vi "PrimeMode API.vi"(8 "error in (no error)":errorcluster, 10 "Pre Purge API Data":T1={"Interval (s)"=0.1, "PurgeDuration (s)"=0.1, "Repeats"=0, "PrimingMode"=enum."Pre-Purge", "Head"=enum."1"}, 11 "TopLevel in":refnum<class "TopLevel.lvclass">) -> (0 "error out":errorcluster, 3 "TopLevel out":refnum<class "TopLevel.lvclass">)   [LabVIEW 2022 SP3, in "TopLevel.lvclass"]
uses:
  TopLevel.lvclass
  Typedefs/PrimingMode APIData.ctl
  Typedefs/PurgeMode--Enum.ctl
  Typedefs/PrinterHeads--Enum.ctl
  Typedefs/API Command Cluster.ctl
  Typedefs/API Command Enum.ctl
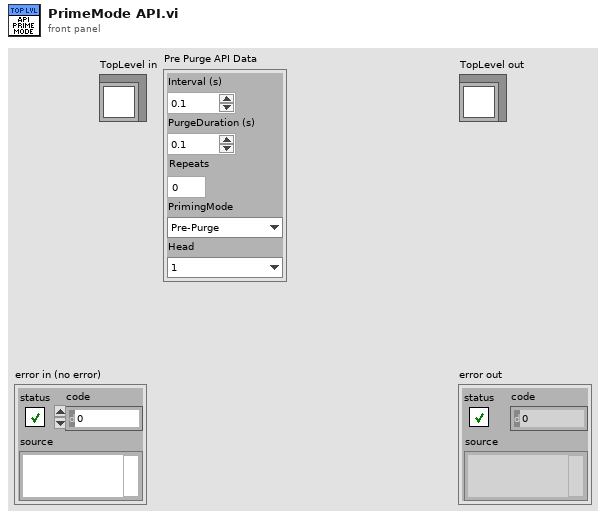
[diagram p1: front panel]
types:
  T1 = typedef "TopLevel.lvclass/PrimingMode APIData.ctl" = cluster{"Interval (s)":dbl, "PurgeDuration (s)":dbl, "Repeats":u8, "PrimingMode":T2, "Head":T3}
  T2 = typedef "PurgeMode--Enum.ctl" = enum16{"Pre-Purge", "Purge", "Spit", "Prime"}
  T3 = typedef "PrinterHeads--Enum.ctl" = enum16{"1", "2", "3", "4", "5", "6", "-1"}
  T4 = typedef "TopLevel.lvclass/API Command Enum.ctl" = enum16{"Execute Printer Commands", "Pre Purge", "Enable Ink Ch-1", "Enable Ink Ch-2", "Enable Ink Ch-3", "Enable Ink Ch-4", "Enable Ink Ch-5", "Enable Ink Ch-6", "Disable Ink Ch-1", "Disable Ink Ch-2", "Disable Ink Ch-3", "Disable Ink Ch-4", "Disable Ink Ch-5", "Disable Ink Ch-6", "ExecuteIdlePrintCycle", "StopIdlePrintCycle", "Abort", "LoadDLP2GUIConfig", "SaveDLP2GUIConfig", "PrimingMode", "SetHeadTemperature", "EnableHead", "EnableHeadHeat", "SetSystemMode", "HeadPrint"}
  T5 = typedef "TopLevel.lvclass/API Command Cluster.ctl" = cluster{"Command":T4, "Arguments":string, "Data":variant}
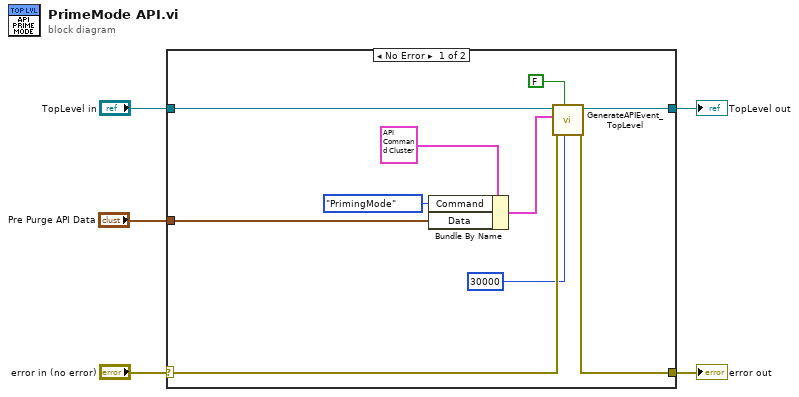
[diagram p0: block diagram]
diagram:
  n1 = case shown="No Error" "error in (no error)" {
    selector: "error in (no error)" -> [w13 w17]
    tunnel: [w12 w17] -> w4
    tunnel: [w15 w16] -> w2
    tunnel: "TopLevel in" -> [w14 w16]
    tunnel: "Pre Purge API Data" -> [w6 _]
    frame No Error {
      n2 = Bundle By Name(cluster=T5 {"Command"=enum."Execute Printer Commands", "Arguments"="", "Data"=variant} ("API Command Cluster"), "Command"=API_Command_Enum."PrimingMode", "Data"=w6) -> (w9:T5)
      n3 = call-dynamic "GenerateAPIEvent_TopLevel.vi"("Timeout (ms)"=u32 30000, "Wait (F)"=FALSE, "error in (no error)"=w13, "API Command Cluster"=w9, "TopLevel in"=w14) -> ("error out"=w12:errorcluster, "TopLevel out"=w15:refnum<class "TopLevel.lvclass">)  [unwired: 5 in]
    }
    frame Error {
    }
  }
  "error out" <- w4
  "TopLevel out" <- w2
